vi "MoveBlock.vi"(0 "srcPointer":u64, 1 "size":u32, 3 "destination":i16[](array[numeric]), 5 "error in (no error)":errorcluster) -> (14 "srcPointer":u64, 15 "size":u32, 17 "destination":i16[](array[numeric]), 19 "error out":errorcluster)   [LabVIEW 2022 SP3, in "Memory.lvlib"]
uses:
  Memory.lvlib
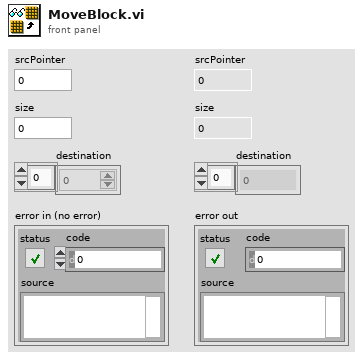
[diagram p1: front panel]
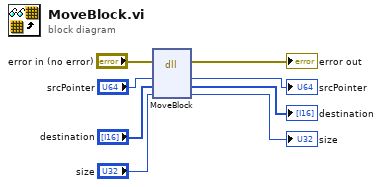
[diagram p0: block diagram]
diagram:
  n1 = dll-call lib="LabVIEW" fn="MoveBlock"(error in="error in (no error)", "Source"="srcPointer", "Destination"="destination", "Size"="size") -> (error out=→"error out":errorcluster, "Source"=→"srcPointer":u64, "Destination"=→"destination":i16[], "Size"=→"size":u32)  [unwired: 3 in, 1 out]
